vi "Agilent 3352X Series Standard Waveform.vi"() -> ()   [LabVIEW 2019]
doc: "This example shows how to generate a standard waveform."
uses:
  Agilent 3352X Series.lvlib
panel:
  in  "DC Offset (0 V)":dbl
  in  "Waveform Function (0: Sine)":u16(ring) items=["Sine"=0, "Square"=1, "Ramp"=2, "Noise"=3, "DC"=4, "Triangle"=5, "Pulse"=6, "Sinc"=11, "D-Lorentz"=12, "Gaussian"=13, "Expo Fall"=14, "Expo Rise"=15, "Haversine"=16]
  in  "Frequency/Sample Rate/Bandwidth (1000 Hz)":dbl=1000.0 format="%#.4f"
  in  "Amplitude (0.1 Vpp)":dbl=0.1
  in  "VISA resource name":refnum<visa-resource-name>
  # "(c) 2011-2021 National Instruments.  ALL RIGHTS RESERVED."
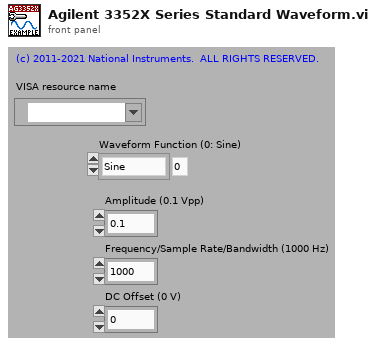
[diagram p1: front panel]
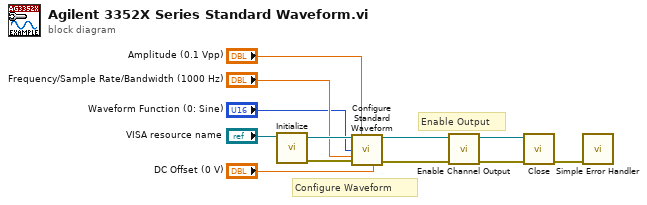
[diagram p0: block diagram]
diagram:
  # "Enable Output"
  # "Configure Waveform"
  n1 = call "Initialize.vi"("VISA resource name"="VISA resource name") -> ("error out"=w6:errorcluster, "VISA resource name out"=w5:refnum<visa-resource-name>)  [unwired: 4 in, 5 out]
  n2 = call "Configure Standard Waveform.vi"("VISA resource name"=w5, "Amplitude (0.1 Vpp)"="Amplitude (0.1 Vpp)", "Waveform Function (0: Sine)"="Waveform Function (0: Sine)", "Frequency/Sample Rate/Bandwidth (1000 Hz)"="Frequency/Sample Rate/Bandwidth (1000 Hz)", "error in (no error)"=w6, "DC Offset (0 V)"="DC Offset (0 V)") -> ("VISA resource name out"=w8:refnum<visa-resource-name>, "error out"=w7:errorcluster)  [unwired: 4 in, 4 out]
  n3 = call "Enable Channel Output.vi"("error in (no error)"=w7, "VISA resource name"=w8) -> ("error out"=w9:errorcluster, "VISA resource name out"=w10:refnum<visa-resource-name>)  [unwired: 3 in, 5 out]
  n4 = call "Close.vi"("error in (no error)"=w9, "VISA resource name"=w10) -> ("error out"=w11:errorcluster)  [unwired: 9 out]
  n5 = call <vilib>:"Simple Error Handler.vi"("error in (no error)"=w11) -> ()  [unwired: 1 in, 8 out]
